vi "PFC Settings Dialog.vi"(8 "error in (no error)":errorcluster, 11 "Ctrl settings in":T1={"FSM status"=enum."Running", "Voltage control ena"=FALSE, "Vea"=16.0, "Voltage Ctrl bypass"=FALSE, "PI Voltage control"={"Ref_val"=0.0, "Kp"=0.0, "Ti"=0.0, "Out_min"=0.0, "Out_max"=0.0}, "Current Ctrl bypass"=FALSE, "PI Current control"={"Ref_val"=0.0, "Kp"=100.0, "Ti"=0.01, "Out_min"=-250.0, "Out_max"=250.0}, "3rd Harmonic"=FALSE, "Output enable"=TRUE}) -> (0 "error out":errorcluster, 1 "Cancelled?":bool, 2 "UI Refresh Needed?":bool, 3 "Ctrl settings out":T1={"FSM status"=enum."Running", "Voltage control ena"=FALSE, "Vea"=6.0, "Voltage Ctrl bypass"=FALSE, "PI Voltage control"={"Ref_val"=0.0, "Kp"=0.0, "Ti"=0.0, "Out_min"=0.0, "Out_max"=0.0}, "Current Ctrl bypass"=FALSE, "PI Current control"={"Ref_val"=0.0, "Kp"=100.0, "Ti"=0.01, "Out_min"=-250.0, "Out_max"=250.0}, "3rd Harmonic"=FALSE, "Output enable"=TRUE})   [LabVIEW 2015, in "Settings.lvlib"]
doc: "Dialog for selecting user specified settings."
uses:
  Settings.lvlib
  PFC Control settings.ctl
  Acquisition/PI Compensator.ctl
panel:
  in  "V_ref":sgl=26.0 caption="Pref"
  in  "V_ctrl byp":bool caption="Bypass (Ref to Vea)"
  in  "V_Lim":sgl=250.0 caption="+/- Lim"
  in  "V_Kp":sgl=100.0 caption="Kp"
  in  "V_Ki2":sgl=0.01 caption="Ti"
  in  "I_ctrl byp":bool caption="Bypass (Ref to d)"
  in  "I_Lim":sgl=250.0 caption="+/- Lim"
  in  "I_Kp":sgl=100.0 caption="Kp"
  in  "I_Ki2":sgl=0.01 caption="Ti"
  in  "3rd harm":bool caption="Third harmonic inj."
  in  "Driver ena":bool=TRUE caption="Driver enable"
  in  "Cancel Button":bool
  in  "Apply Button":bool
  # "Non visible portion of dialog (needed for connector pane)."
  # "da"
  # "Alfa Ref"
  # "Vea"
  # "db"
  # "Beta Ref"
  # "dc"
  # "VDC out"
  # "Voltage Control"
  # "VLa"
  # "VLb"
  # "VLc"
  # "Current Reference \nGenerator"
  # "ILa"
  # "ILb"
  # "ILc"
  # "PWM Generation"
  # "Current Control"
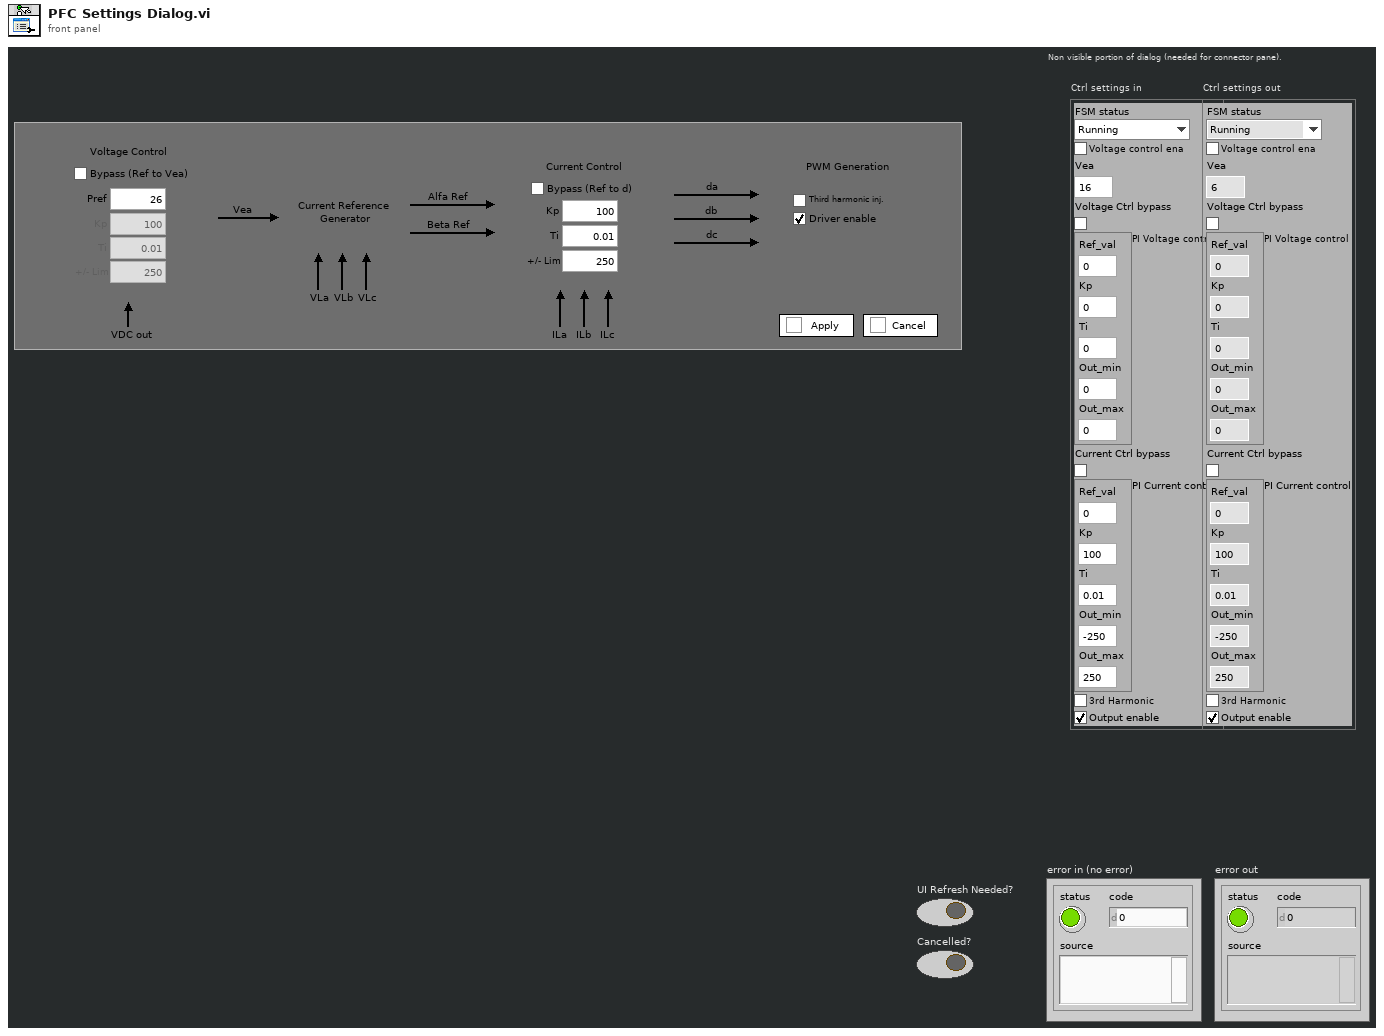
[diagram p1: front panel]
types:
  T1 = typedef "Settings.lvlib/PFC Control settings.ctl" = cluster{"FSM status":enum8{"Stopped", "Running"}, "Voltage control ena":bool, "Vea":sgl, "Voltage Ctrl bypass":bool, "PI Voltage control":T2, "Current Ctrl bypass":bool, "PI Current control":T2, "3rd Harmonic":bool, "Output enable":bool}
  T2 = typedef "Settings.lvlib/PI Compensator.ctl" = cluster{"Ref_val":sgl, "Kp":sgl, "Ti":sgl, "Out_min":sgl, "Out_max":sgl}
  T3 = enum8{"Enabled", "Disabled", "Disabled and Grayed Out"}
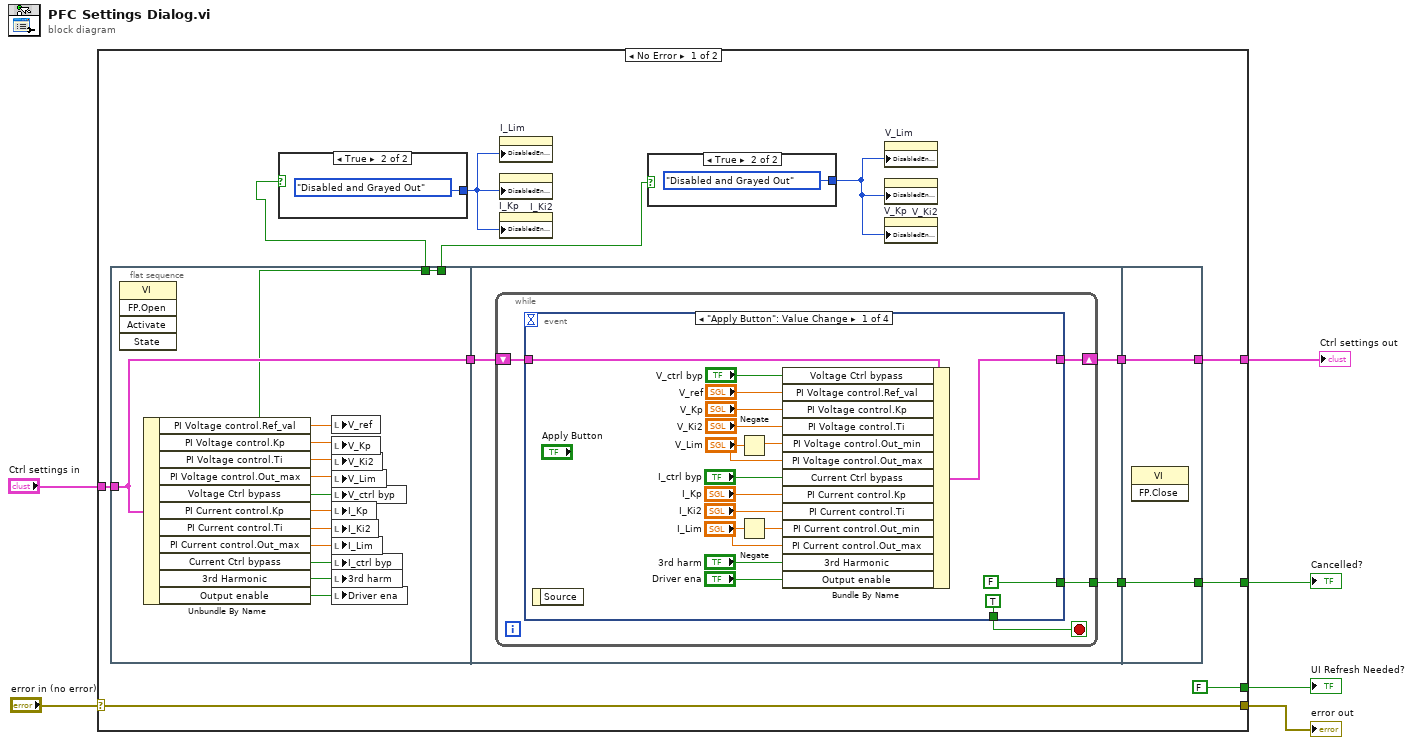
[diagram p0: block diagram]
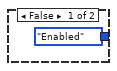
[diagram p2: hidden frame]
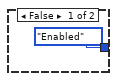
[diagram p3: hidden frame]
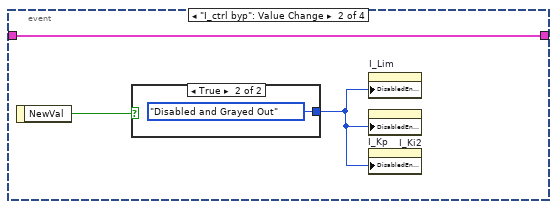
[diagram p4: hidden frame]
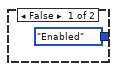
[diagram p5: hidden frame]
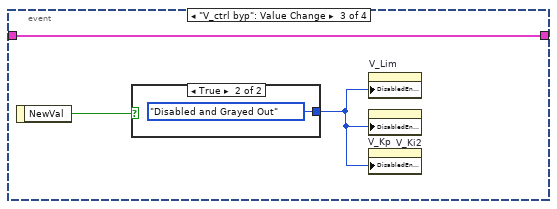
[diagram p6: hidden frame]
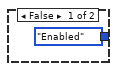
[diagram p7: hidden frame]
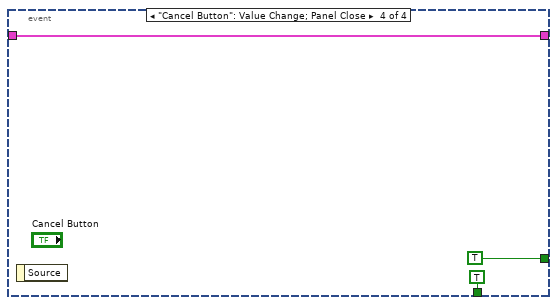
[diagram p8: hidden frame]
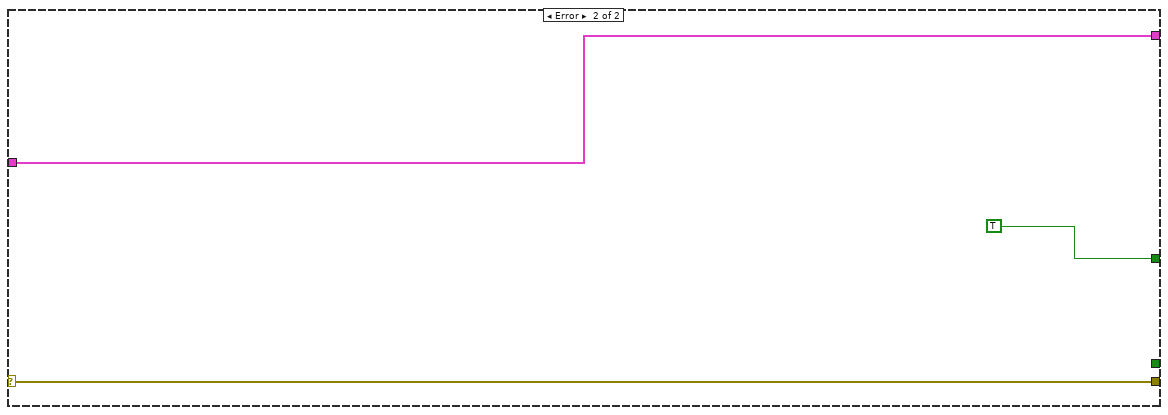
[diagram p9: hidden frame]
diagram:
  n1 = case shown="No Error" "error in (no error)" {
    selector: "error in (no error)" -> [w18 w76]
    tunnel: [w18 w76] -> w5
    tunnel: "Ctrl settings in" -> [w14 w75]
    tunnel: [w15 w75] -> w2
    tunnel: [FALSE ("UI Refresh Needed?") _] -> w4
    tunnel: [w16 TRUE ("UI Refresh Needed?")] -> w3
    frame No Error {
      n2 = flat-sequence {
        tunnel: w14 -> [w29]
        tunnel: [w29] -> w10
        tunnel: [w24] -> w8
        tunnel: [w23] -> w7
        tunnel: [w37] -> w13
        tunnel: [w36] -> w12
        tunnel: w10 -> [w35]
        tunnel: [w72] -> w15
        tunnel: [w73] -> w16
        tunnel: w13 -> [w73]
        tunnel: w12 -> [w72]
        frame #0 {
          n3 = invoke class="VI" method="FP.Open"() -> ()  [unwired: 5 in, 5 out]
          n4 = Unbundle By Name(w29) -> ("PI Voltage control.Ref_val"=w28:sgl, "PI Voltage control.Kp"=w26:sgl, "PI Voltage control.Ti"=w27:sgl, "PI Voltage control.Out_max"=w25:sgl, "Voltage Ctrl bypass"=w23:bool, "PI Current control.Kp"=w32:sgl, "PI Current control.Ti"=w33:sgl, "PI Current control.Out_max"=w34:sgl, "Current Ctrl bypass"=w24:bool, "3rd Harmonic"=w31:bool, "Output enable"=w30:bool)
          n5 = local write "V_ref"(w28) -> ()
          n6 = local write "V_Kp"(w26) -> ()
          n7 = local write "V_Ki2"(w27) -> ()
          n8 = local write "V_Lim"(w25) -> ()
          n9 = local write "V_ctrl byp"(w23) -> ()
          n10 = local write "I_Kp"(w32) -> ()
          n11 = local write "I_Ki2"(w33) -> ()
          n12 = local write "I_Lim"(w34) -> ()
          n13 = local write "I_ctrl byp"(w24) -> ()
          n14 = local write "3rd harm"(w31) -> ()
          n15 = local write "Driver ena"(w30) -> ()
        }
        frame #1 {
          n16 = while {
            tunnel: [w41] -> w37
            shift-right: [w40] -> w36
            shift-left: w35 -> [w39]
            stop <- w38 stop-if-true
            n17 = event shown="[0] \"Apply Button\": Value Change" {
              selector: _ -> [_ _ _ _]
              dyn-events: _ -> [_ _ _ _]
              timeout: _ -> [_ _ _ _]
              tunnel: [w56 w61 w66 w71] -> w40
              tunnel: w39 -> [w57 w61 w66 w71]
              tunnel: [FALSE ("UI Refresh Needed?") _ _ TRUE ("UI Refresh Needed?")] -> w41
              tunnel: [TRUE ("UI Refresh Needed?") _ _ TRUE ("UI Refresh Needed?")] -> w38
              event "Apply Button": Value Change {
                n18 = event-data() -> ()  [unwired: 1 in, 1 out]
                n19 = Negate(x="V_Lim") -> (-x=w47:sgl)
                n20 = Negate(x="I_Lim") -> (-x=w50:sgl)
                n21 = Bundle By Name(cluster=w57, "Voltage Ctrl bypass"="V_ctrl byp", "PI Voltage control.Ref_val"="V_ref", "PI Voltage control.Kp"="V_Kp", "PI Voltage control.Ti"="V_Ki2", "PI Voltage control.Out_min"=w47, "PI Voltage control.Out_max"="V_Lim", "Current Ctrl bypass"="I_ctrl byp", "PI Current control.Kp"="I_Kp", "PI Current control.Ti"="I_Ki2", "PI Current control.Out_min"=w50, "PI Current control.Out_max"="I_Lim", "3rd Harmonic"="3rd harm", "Output enable"="Driver ena") -> (w56:T1)
              }
              event "I_ctrl byp": Value Change {
                n22 = event-data() -> ("NewVal"=w59:bool)  [unwired: 1 in]
                n23 = case shown="True" w59 {
                  tunnel: [T3."Enabled" ("Disabled") T3."Disabled and Grayed Out" ("Disabled")] -> w60
                  frame False {
                  }
                  frame True {
                  }
                }
                n24 = property on="I_Lim" class="DigNum (strict)"("DisabledEnum"=w60) -> ()  [unwired: 2 in, 2 out]
                n25 = property on="I_Ki2" class="DigNum (strict)"("DisabledEnum"=w60) -> ()  [unwired: 2 in, 2 out]
                n26 = property on="I_Kp" class="DigNum (strict)"("DisabledEnum"=w60) -> ()  [unwired: 2 in, 2 out]
              }
              event "V_ctrl byp": Value Change {
                n27 = event-data() -> ("NewVal"=w64:bool)  [unwired: 1 in]
                n28 = case shown="True" w64 {
                  tunnel: [T3."Enabled" ("Disabled") T3."Disabled and Grayed Out" ("Disabled")] -> w65
                  frame False {
                  }
                  frame True {
                  }
                }
                n29 = property on="V_Lim" class="DigNum (strict)"("DisabledEnum"=w65) -> ()  [unwired: 2 in, 2 out]
                n30 = property on="V_Ki2" class="DigNum (strict)"("DisabledEnum"=w65) -> ()  [unwired: 2 in, 2 out]
                n31 = property on="V_Kp" class="DigNum (strict)"("DisabledEnum"=w65) -> ()  [unwired: 2 in, 2 out]
              }
              event "Cancel Button": Value Change; Panel Close {
                n32 = event-data() -> ()  [unwired: 1 in, 1 out]
              }
            }
          }
        }
        frame #2 {
          n33 = invoke class="VI" method="FP.Close"() -> ()  [unwired: 3 in, 3 out]
        }
      }
      n34 = case shown="True" w8 {
        tunnel: [T3."Enabled" ("Disabled") T3."Disabled and Grayed Out" ("Disabled")] -> w11
        frame False {
        }
        frame True {
        }
      }
      n35 = property on="I_Lim" class="DigNum (strict)"("DisabledEnum"=w11) -> ()  [unwired: 2 in, 2 out]
      n36 = property on="I_Ki2" class="DigNum (strict)"("DisabledEnum"=w11) -> ()  [unwired: 2 in, 2 out]
      n37 = property on="I_Kp" class="DigNum (strict)"("DisabledEnum"=w11) -> ()  [unwired: 2 in, 2 out]
      n38 = case shown="True" w7 {
        tunnel: [T3."Enabled" ("Disabled") T3."Disabled and Grayed Out" ("Disabled")] -> w9
        frame False {
        }
        frame True {
        }
      }
      n39 = property on="V_Lim" class="DigNum (strict)"("DisabledEnum"=w9) -> ()  [unwired: 2 in, 2 out]
      n40 = property on="V_Ki2" class="DigNum (strict)"("DisabledEnum"=w9) -> ()  [unwired: 2 in, 2 out]
      n41 = property on="V_Kp" class="DigNum (strict)"("DisabledEnum"=w9) -> ()  [unwired: 2 in, 2 out]
    }
    frame Error {
    }
  }
  "UI Refresh Needed?" <- w4
  "error out" <- w5
  "Cancelled?" <- w3
  "Ctrl settings out" <- w2
